vi "Data_Modifier_Client.vi"() -> ()   [LabVIEW 2021]
panel:
  in  "Stop":bool
  in  "Data in 2":string
  out "Data out":string
  in  "Send":bool
  out "error out":errorcluster
  in  "error in (no error)":errorcluster
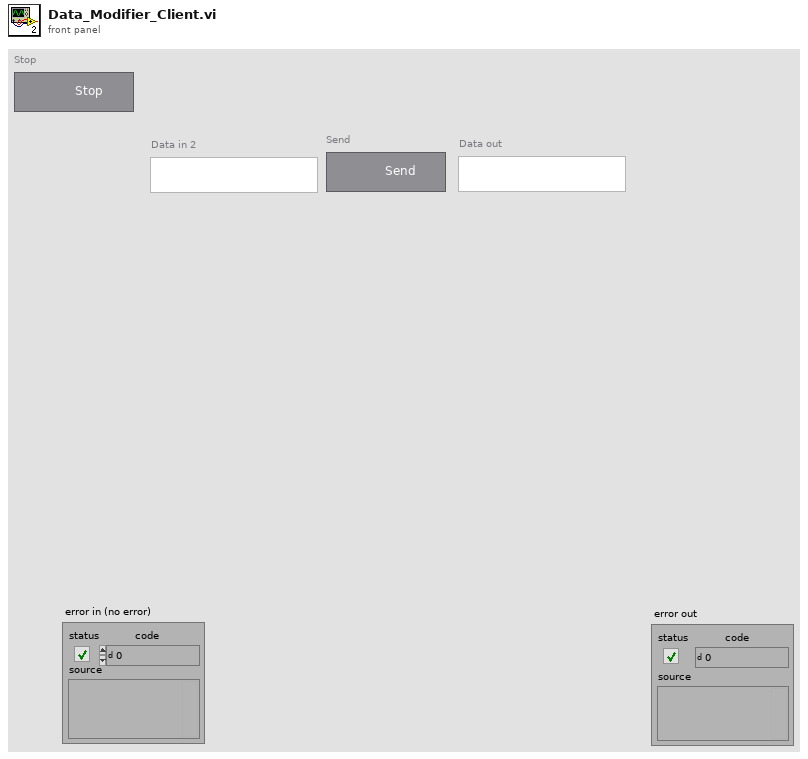
[diagram p1: front panel]
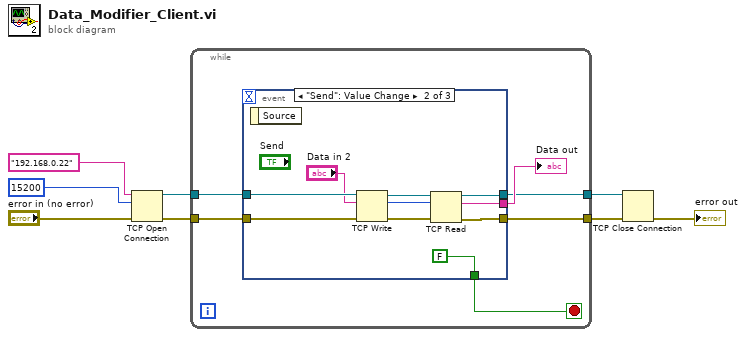
[diagram p0: block diagram]
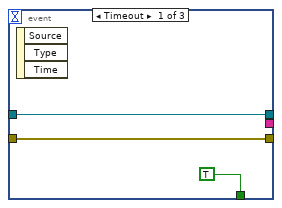
[diagram p2: hidden frame]
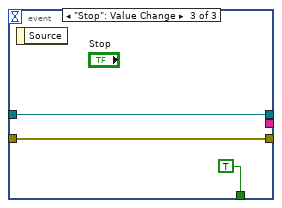
[diagram p3: hidden frame]
diagram:
  n1 = TCP Open Connection(address="192.168.0.22", remote port or service name=u16 15200, error in (no error)="error in (no error)") -> (connection ID=w5:refnum<k5>, error out=w6:errorcluster)  [unwired: 2 in]
  n2 = while {
    tunnel: w5 -> [w13]
    tunnel: w6 -> [w14]
    tunnel: [w10] -> w3
    tunnel: [w9] -> w1
    stop <- w12 stop-if-true
    n3 = event shown="[1] \"Send\": Value Change" {
      selector: _ -> [_ _ _]
      dyn-events: _ -> [_ _ _]
      timeout: _ -> [_ _ _]
      tunnel: w14 -> [w17 w27 w30]
      tunnel: w13 -> [w15 w26 w28]
      tunnel: [_ w23 _] -> w11
      tunnel: [w17 w22 w30] -> w10
      tunnel: [TRUE FALSE TRUE] -> w12
      tunnel: [w15 w18 w28] -> w9
      event Timeout {
        n4 = event-data() -> ()  [unwired: 1 in, 3 out]
      }
      event "Send": Value Change {
        n5 = event-data() -> ()  [unwired: 1 in, 1 out]
        n6 = TCP Write(connection ID=w26, data in="Data in 2", error in (no error)=w27) -> (connection ID out=w24:refnum<k5>, bytes written=w20:i32, error out=w25:errorcluster)  [unwired: 1 in]
        n7 = TCP Read(connection ID=w24, bytes to read=w20, error in (no error)=w25) -> (connection ID out=w18:refnum<k5>, data out=w23:string, error out=w22:errorcluster)  [unwired: 2 in]
      }
      event "Stop": Value Change {
        n8 = event-data() -> ()  [unwired: 1 in, 1 out]
      }
    }
    "Data out" <- w11
  }
  n9 = TCP Close Connection(connection ID=w1, error in (no error)=w3) -> (error out=→"error out":errorcluster)  [unwired: 1 in, 1 out]
